vi "Open.vi"(0 "reference in":refnum<class "TimedDoor.lvclass">, 5 "error in (no error)":errorcluster) -> (14 "reference out":refnum<class "TimedDoor.lvclass">, 19 "error out":errorcluster)   [LabVIEW 2020, in "TimedDoor.lvclass"]
uses:
  TimedDoor.lvclass
  TimedDoor.lvclass/TimedDoor.ctl
  Door_class/Door.lvclass
  LcTimer_class/LcTimer.lvclass
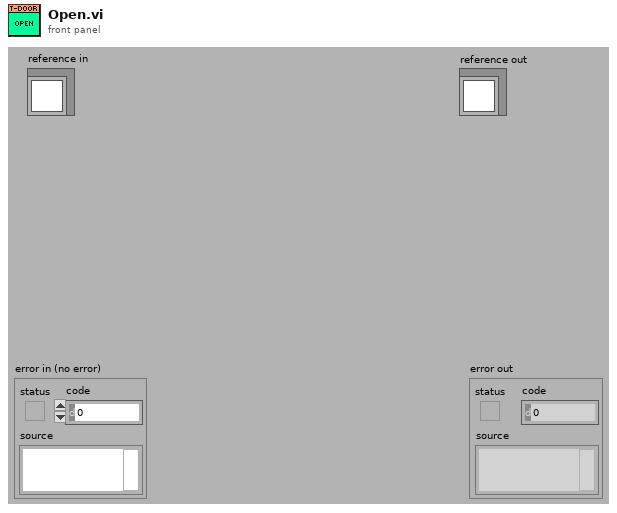
[diagram p1: front panel]
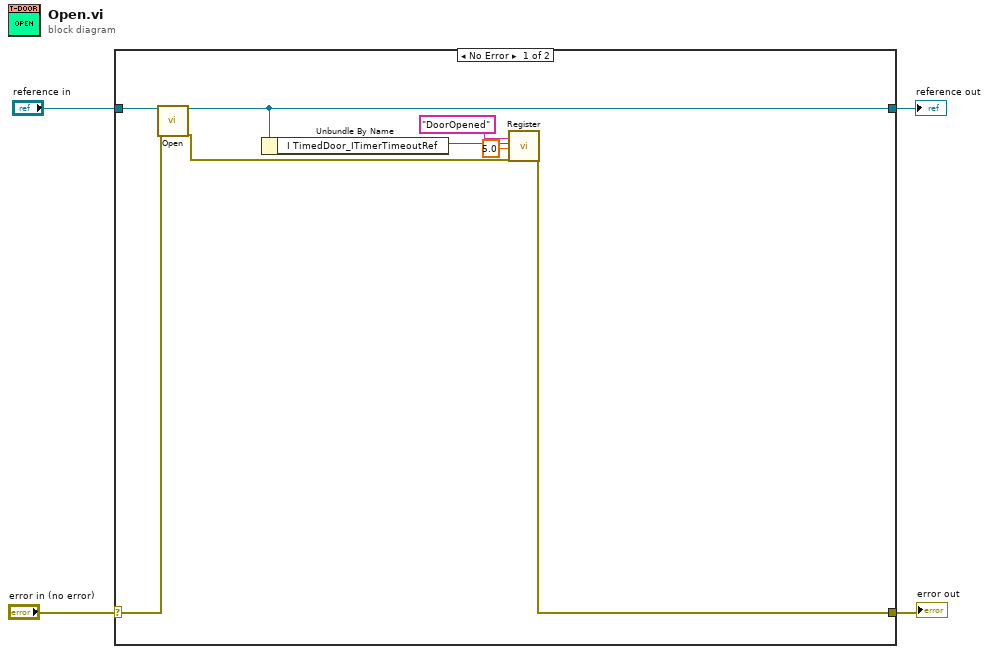
[diagram p0: block diagram]
diagram:
  n1 = case shown="No Error" "error in (no error)" {
    selector: "error in (no error)" -> [w11 w14]
    tunnel: [w5 w14] -> w3
    tunnel: [w10 w13] -> w1
    tunnel: "reference in" -> [w12 w13]
    frame No Error {
      n2 = call-parent "Open.vi"("reference in"=w12, "error in (no error)"=w11) -> ("reference out"=w10:refnum<class "TimedDoor.lvclass">, "error out"=w6:errorcluster)  [unwired: 16 in]
      n3 = Unbundle By Name(w10) -> ("I TimedDoor_ITimerTimeoutRef"=w9:refnum<class "ITimerTimeout.lvclass">)
      n4 = call "Register.vi"("TimeoutName"="DoorOpened", "TimeoutInterface"=w9, "TimeoutTime(s)"=5.0, "error in (no error)"=w6) -> ("error out"=w5:errorcluster)  [unwired: 14 in, 1 out]
    }
    frame Error {
    }
  }
  "error out" <- w3
  "reference out" <- w1
